vi "Receive.vi"(8 "error in":errorcluster, 10 "Transfer Group in":refnum<class "Transfer Group.lvclass">, 11 "RDMA Transceiver in":refnum<class "RDMA Transceiver.lvclass">) -> (0 "error out":errorcluster, 2 "Transfer Group out":refnum<class "Transfer Group.lvclass">, 3 "RDMA Transceiver out":refnum<class "RDMA Transceiver.lvclass">)   [LabVIEW 2020, in "RDMA.lvlib" / "RDMA Transceiver.lvclass"]
doc: "Fetches data over RDMA and writes this data to DSF buffers."
uses:
  RDMA Transceiver.lvclass
  DSF Core.lvlibp/Classes/Transfer Group/Transfer Group.lvclass
  RDMA Transceiver.lvclass/RDMA Transceiver.ctl
  Read From RDMA Buffer.vi
  <vilib>/Utility/error.llb/Clear Errors.vi
  <vilib>/rdma/rdma.llb/RDMA Acquire Received Buffer.vi
  <vilib>/rdma/rdma.llb/RDMA Acquire Received Buffer U8.vi
  DSF Core.lvlibp/Classes/Transfer/Get Active Buffer.vi
  DSF Core.lvlibp/Classes/Buffer/Get Buffer Size.vi
  Throw Error.vi
  Throw Size Mismatch Error.vi
  DSF Core.lvlibp/Classes/Buffer/Write Buffer.vi
  DSF Core.lvlibp/Classes/Buffer/Write Buffer 1D U8.vi
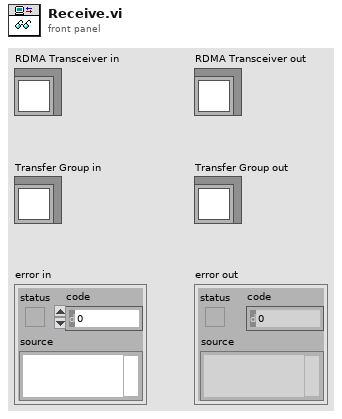
[diagram p1: front panel]
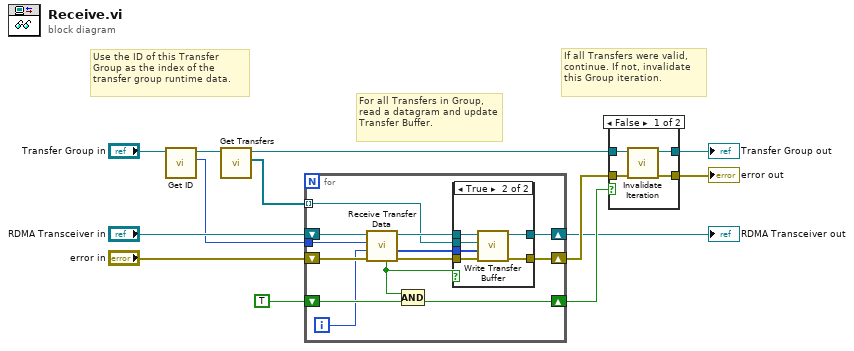
[diagram p0: block diagram]
diagram:
  # "If all Transfers were valid, continue. If not, invalidate this Group iteration."
  # "Use the ID of this Transfer Group as the index of the transfer group runtime data."
  # "For all Transfers in Group, read a datagram and update Transfer Buffer."
  n1 = call "Get ID.vi"("Transfer Group in"="Transfer Group in") -> ("id"=w3:i32, "Transfer Group out"=w13:refnum<class "Transfer Group.lvclass">)  [unwired: 9 in]
  n2 = call "Get Transfers.vi"("Transfer Group in"=w13) -> ("Transfers"=w4:refnum<class "Transfer.lvclass">[], "Transfer Group out"=w6:refnum<class "Transfer Group.lvclass">)  [unwired: 9 in]
  n3 = for {
    shift-right: [w20] -> w11
    shift-left: "error in" -> [w25]
    shift-right: [w21] -> w2
    shift-left: "RDMA Transceiver in" -> [w26]
    tunnel: w3 -> [w17]
    shift-right: [w18] -> w7
    shift-left: TRUE -> [w19]
    tunnel: w4 -> [w15] mode=indexing
    i -> [w16]
    n4 = call "Receive Transfer Data.vi"("error in"=w25, "transfer id"=w16, "transfer group id"=w17, "RDMA Transceiver in"=w26) -> ("error out"=w23:errorcluster, "transfer data"=w22:u8[], "RDMA Transceiver out"=w24:refnum<class "RDMA Transceiver.lvclass">, "valid"=w14:bool)  [unwired: 4 in]
    n5 = Compound Arithmetic op=AND(w14, w19) -> (w18:bool)
    n6 = case shown="True" w14 {
      tunnel: w24 -> [w28 w34]
      tunnel: w23 -> [w27 w33]
      tunnel: w22 -> [_ w32]
      tunnel: [w28 w31] -> w21
      tunnel: [w27 w30] -> w20
      tunnel: w15 -> [_ w29]
      frame False {
      }
      frame True {
        n7 = call "Write Transfer Buffer.vi"("error in"=w33, "data"=w32, "Transfer"=w29, "RDMA Transceiver in"=w34) -> ("error out"=w30:errorcluster, "RDMA Transceiver out"=w31:refnum<class "RDMA Transceiver.lvclass">)  [unwired: 6 in]
      }
    }
  }
  "RDMA Transceiver out" <- w2
  n8 = case shown="False" w7 {
    tunnel: w11 -> [w38 w40]
    tunnel: [w37 w40] -> w1
    tunnel: w6 -> [w36 w39]
    tunnel: [w35 w39] -> w5
    frame False {
      n9 = call "Invalidate Iteration.vi"("error in (no error)"=w38, "Transfer Group in"=w36) -> ("error out"=w37:errorcluster, "Transfer Group out"=w35:refnum<class "Transfer Group.lvclass">)  [unwired: 8 in]
    }
    frame True {
    }
  }
  "error out" <- w1
  "Transfer Group out" <- w5
